vi "IrInitializeQbus.vi"(8 "error in (no error)":errorcluster) -> (0 "error out":errorcluster, 3 "Qbus out":refnum<class "Qbus.lvclass">)   [LabVIEW 2017]
uses:
  <vilib>/addons/Qbus/Qbus.lvclass
  <vilib>/addons/BlinkProcess/BlinkProcess.lvlib
  <vilib>/addons/TimerProcess/TimerProcess.lvlib
  <vilib>/addons/InsightCM/Devices/Shared/Common/ServerComm/ServerComm.lvlib
  <vilib>/addons/InsightCM/Devices/Shared/Common/Trigger/Trigger.lvlib
  <vilib>/addons/TraceLogger/TraceLogger.lvlib
  <vilib>/addons/InsightCM/Devices/Shared/Common/FileManager/FileManager.lvlib
  <vilib>/addons/InsightCM/Devices/Shared/Common/Controller/Controller.lvlib
  <vilib>/addons/InsightCM/Devices/Shared/Common/DeviceHealth/DeviceHealth.lvlib
  <vilib>/addons/InsightCM/Devices/Shared/Ir/IrAnalysis/IrAnalysis.lvlib
  <vilib>/addons/InsightCM/Devices/Shared/Ir/IrAcquisition/IrAcquisition.lvlib
  <vilib>/addons/InsightCM/Devices/Shared/Ir/IrManageCameras/IrManageCameras.lvlib
  <vilib>/addons/InsightCM/Devices/Shared/Common/TrendAlarm/TrendAlarm.lvlib
  <vilib>/addons/InsightCM/Devices/Shared/Ir/IrDataEventCreator/IrDataEventCreator.lvlib
  <vilib>/addons/InsightCM/Devices/Shared/Ir/IrTestPanel/IrTestPanel.lvlib
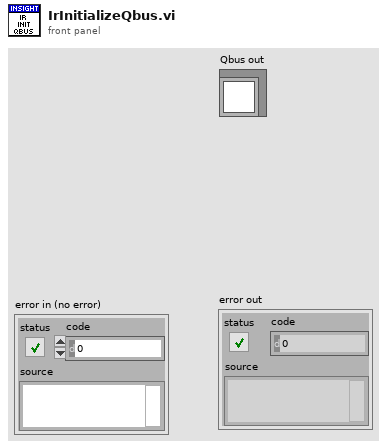
[diagram p1: front panel]
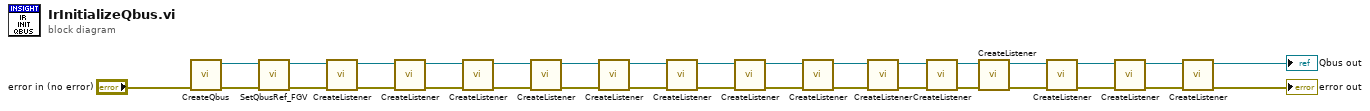
[diagram p0: block diagram]
diagram:
  n1 = call <vilib>:"CreateQbus.vi"("error in (no error)"="error in (no error)") -> ("error out"=w24:errorcluster, "Qbus"=w23:refnum<class "Qbus.lvclass">)  [unwired: 9 in]
  n2 = call <vilib>:"SetQbusRef_FGV.vi"("error in (no error)"=w24, "Qbus in"=w23) -> ("error out"=w22:errorcluster, "Qbus out"=w21:refnum<class "Qbus.lvclass">)  [unwired: 8 in]
  n3 = call <vilib>:"CreateListener.vi"("error in (no error)"=w22, "Qbus in"=w21) -> ("error out"=w26:errorcluster, "Qbus out"=w25:refnum<class "Qbus.lvclass">)  [unwired: 8 in]
  n4 = call <vilib>:"CreateListener.vi"("error in (no error)"=w26, "Qbus in"=w25) -> ("error out"=w12:errorcluster, "Qbus out"=w11:refnum<class "Qbus.lvclass">)  [unwired: 8 in]
  n5 = call <vilib>:"CreateListener.vi"("error in (no error)"=w12, "Qbus in"=w11) -> ("error out"=w27:errorcluster, "Qbus out"=w28:refnum<class "Qbus.lvclass">)  [unwired: 8 in]
  n6 = call <vilib>:"CreateListener.vi"("error in (no error)"=w27, "qbus in"=w28) -> ("error out"=w13:errorcluster, "qbus out"=w14:refnum<class "Qbus.lvclass">)  [unwired: 8 in]
  n7 = call <vilib>:"CreateListener.vi"("error in (no error)"=w13, "Qbus in"=w14) -> ("error out"=w16:errorcluster, "Qbus out"=w15:refnum<class "Qbus.lvclass">)  [unwired: 8 in]
  n8 = call <vilib>:"CreateListener.vi"("error in (no error)"=w16, "Qbus in"=w15) -> ("error out"=w17:errorcluster, "Qbus out"=w18:refnum<class "Qbus.lvclass">)  [unwired: 8 in]
  n9 = call <vilib>:"CreateListener.vi"("error in (no error)"=w17, "Qbus in"=w18) -> ("error out"=w9:errorcluster, "Qbus out"=w10:refnum<class "Qbus.lvclass">)  [unwired: 8 in]
  n10 = call <vilib>:"CreateListener.vi"("error in (no error)"=w9, "Qbus in"=w10) -> ("error out"=w6:errorcluster, "Qbus out"=w5:refnum<class "Qbus.lvclass">)  [unwired: 8 in]
  n11 = call <vilib>:"CreateListener.vi"("error in (no error)"=w6, "Qbus in"=w5) -> ("error out"=w3:errorcluster, "Qbus out"=w4:refnum<class "Qbus.lvclass">)  [unwired: 8 in]
  n12 = call <vilib>:"CreateListener.vi"("error in (no error)"=w3, "Qbus in"=w4) -> ("error out"=w1:errorcluster, "Qbus out"=w2:refnum<class "Qbus.lvclass">)  [unwired: 8 in]
  n13 = call <vilib>:"CreateListener.vi"("error in (no error)"=w1, "Qbus in"=w2) -> ("error out"=w19:errorcluster, "Qbus out"=w20:refnum<class "Qbus.lvclass">)  [unwired: 8 in]
  n14 = call <vilib>:"CreateListener.vi"("error in (no error)"=w19, "Qbus in"=w20) -> ("error out"=w8:errorcluster, "Qbus out"=w7:refnum<class "Qbus.lvclass">)  [unwired: 8 in]
  n15 = call <vilib>:"CreateListener.vi"("error in (no error)"=w8, "Qbus in"=w7) -> ("error out"=w32:errorcluster, "Qbus out"=w33:refnum<class "Qbus.lvclass">)  [unwired: 8 in]
  n16 = call <vilib>:"CreateListener.vi"("error in (no error)"=w32, "qbus in"=w33) -> ("error out"=→"error out":errorcluster, "qbus out"=→"Qbus out":refnum<class "Qbus.lvclass">)  [unwired: 8 in]
